vi "Configure Acquisition Type.vi"(7 "Number Of Averages (8)":i32=8, 8 "error in (no error)":errorcluster, 9 "Acquisition Mode (0: Real time)":i32(ring) items=["Real time ", "Equivalent time"], 10 "Acquisition Type (0: Normal)":i32(ring) items=["Normal", "Average", "Peak Detect"], 11 "VISA resource name":refnum<visa-resource-name>) -> (0 "error out":errorcluster, 3 "VISA resource name out":refnum<visa-resource-name>)   [LabVIEW 2023, in "RIGOL DS1054Z.lvlib"]
doc: "Configures acquisition type of the oscilloscope."
uses:
  RIGOL DS1054Z.lvlib
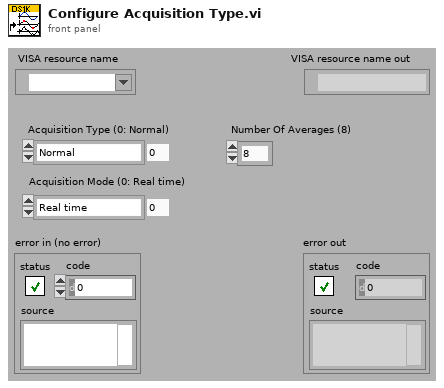
[diagram p1: front panel]
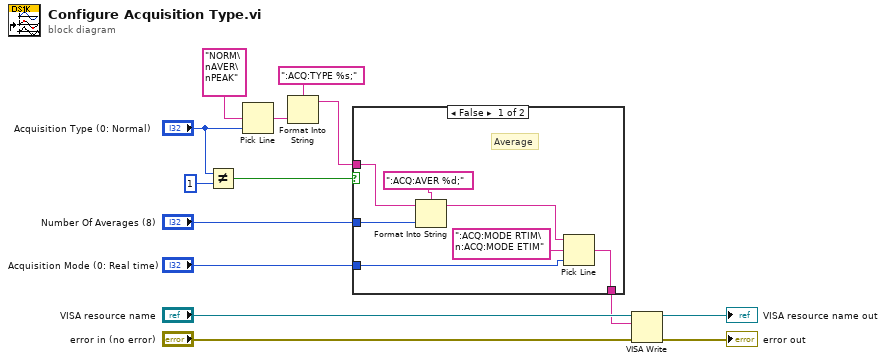
[diagram p0: block diagram]
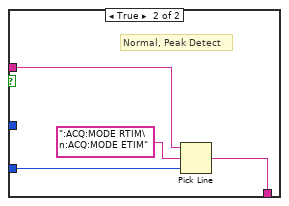
[diagram p2: hidden frame]
diagram:
  n1 = Not Equal?(x="Acquisition Type (0: Normal)", y=1) -> (x != y?=w4:bool)
  n2 = Pick Line(multi-line string="NORM\nAVER\nPEAK", line index="Acquisition Type (0: Normal)") -> (output string=w10:string)  [unwired: 1 out]
  n3 = Format Into String(format string=":ACQ:TYPE %s;", w10) -> (resulting string=w6:string)  [unwired: 2 in, 1 out]
  n4 = case shown="False" w4 {
    tunnel: "Acquisition Mode (0: Real time)" -> [w19 w25]
    tunnel: w6 -> [w16 w24]
    tunnel: [w17 w22] -> w5
    tunnel: "Number Of Averages (8)" -> [w18 _]
    frame False {
      # "Average"
      n5 = Format Into String(format string=":ACQ:AVER %d;", initial string=w16, w18) -> (resulting string=w15:string)  [unwired: 1 in, 1 out]
      n6 = Pick Line(string ("")=w15, multi-line string=":ACQ:MODE RTIM\n:ACQ:MODE ETIM", line index=w19) -> (output string=w17:string)
    }
    frame True {
      # "Normal, Peak Detect"
      n7 = Pick Line(string ("")=w24, multi-line string=":ACQ:MODE RTIM\n:ACQ:MODE ETIM", line index=w25) -> (output string=w22:string)
    }
  }
  n8 = VISA Write(VISA resource name="VISA resource name", write buffer=w5, error in (no error)="error in (no error)") -> (VISA resource name out=→"VISA resource name out":refnum<visa-resource-name>, error out=→"error out":errorcluster)  [unwired: 1 out]
